vi "Over Current Dead Short to VBAT.vi"(3 "error in":errorcluster) -> (10 "error out":errorcluster)   [LabVIEW 2015]
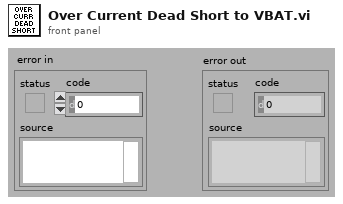
[diagram p1: front panel]
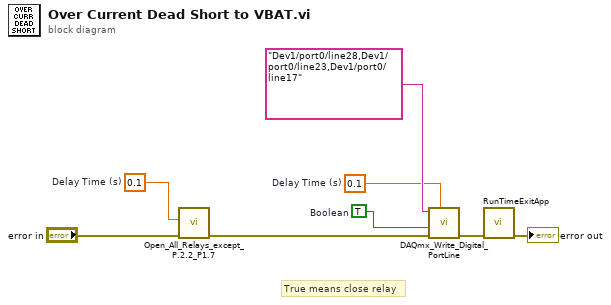
[diagram p0: block diagram]
diagram:
  w1 = 0.1  # Delay Time (s)
  w2 = 0.1  # Delay Time (s)
  w8 = TRUE  # Boolean
  # "True means close relay"
  n1 = call "Open_All_Relays_except_P.2.2_P1.7.vi"("Delay Time (s)"=w1, "error in"="error in") -> ("error out"=w3:errorcluster)  [unwired: 7 in]
  n2 = call "DAQmx_Write_Digital_PortLine.vi"("Device/Ports/Lines"="Dev1/port0/line28,Dev1/port0/line23,Dev1/port0/line17", "Boolean"=w8, "error in"=w3, "Delay Time (s)"=w2) -> ("error out"=w7:errorcluster)  [unwired: 5 in, 1 out]
  n3 = call "RunTimeExitApp.vi"("error in (no error)"=w7) -> ("error out"=→"error out":errorcluster)  [unwired: 10 in]
